vi "Stop Core.vi"(10 "final error code":i32, 11 "Acquisition in":refnum<class "Acquisition.lvclass">) -> (3 "Acquisition out":refnum<class "Acquisition.lvclass">)   [LabVIEW 2020, in "Acquisition.lvlib" / "Acquisition.lvclass"]
doc: "(<B>Filename</B>: Actor Framework.lvlib:Actor.lvclass:Stop Core.vi)\n\nDefines what the actor does before it stops. Use the <B>final error code</B> input to determine whether the actor shut down in response to an error.\n\nBy default, this method passes the Stop message along to all auto-stop nested actors. A descendant class may override this method to define additional behavior, such as shutting down any processes the actor initiated in its override of the Actor Core method."
uses:
  Acquisition.lvclass
  Acquisition.lvclass/Acquisition.ctl
  <vilib>/ActorFramework/Actor/Actor.lvclass
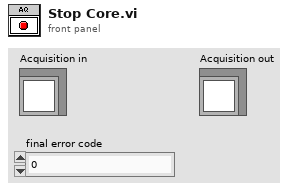
[diagram p1: front panel]
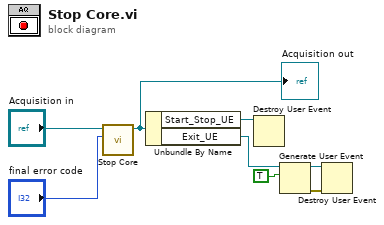
[diagram p0: block diagram]
diagram:
  n1 = call-parent "Stop Core.vi"("final error code"="final error code", "Actor in"="Acquisition in") -> ("Actor out"=w6:refnum<class "Acquisition.lvclass">)  [unwired: 9 in]
  "Acquisition out" <- w6
  n2 = Unbundle By Name(w6) -> ("Start_Stop_UE"=w5:refnum<user-event>, "Exit_UE"=w2:refnum<user-event>)
  n3 = Destroy User Event(user event=w5) -> ()  [unwired: 1 in, 1 out]
  n4 = Generate User Event(user event=w2, event data cluster=TRUE ("event data")) -> (user event out=w3:refnum<user-event>, error out=w4:errorcluster)  [unwired: 2 in]
  n5 = Destroy User Event(user event=w3, error in=w4) -> ()  [unwired: 1 out]
